vi "Set Display Direction.vi"(8 "error in (no error)":errorcluster, 10 "Direction":T1, 11 "senseHatDisplay in":refnum<class "RPI.SenseHat.Display.lvclass">) -> (0 "error out":errorcluster, 3 "senseHatDisplay out":refnum<class "RPI.SenseHat.Display.lvclass">)   [LabVIEW 2020, in "RPI.SenseHat.Display.lvlib" / "RPI.SenseHat.Display.lvclass"]
doc: "Sets new display direction."
uses:
  RPI.SenseHat.Display.lvclass
  TypeDefs/Display Direction.ctl
  RPI.SenseHat.Display.lvclass/RPI.SenseHat.Display.ctl
  RPI.SenseHat.Display.lvlib
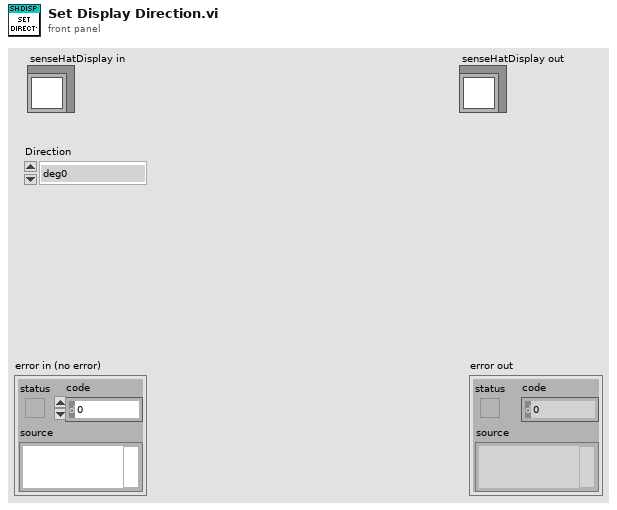
[diagram p1: front panel]
types:
  T1 = typedef "RPI.SenseHat.Display.lvlib/Display Direction.ctl" = enum16{"deg0", "deg90", "deg180", "deg270"}
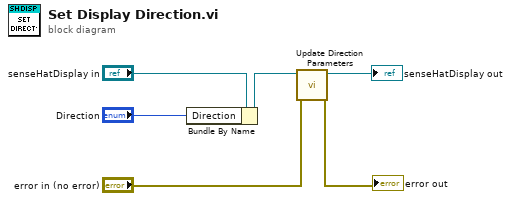
[diagram p0: block diagram]
diagram:
  n1 = Bundle By Name(cluster="senseHatDisplay in", "Direction"="Direction") -> (w4:refnum<class "RPI.SenseHat.Display.lvclass">)
  n2 = call "Update Direction Parameters.vi"("error in (no error)"="error in (no error)", "senseHatDisplay in"=w4) -> ("error out"=→"error out":errorcluster, "senseHatDisplay out"=→"senseHatDisplay out":refnum<class "RPI.SenseHat.Display.lvclass">)  [unwired: 8 in]
